vi "GetEntryGoToItem.vi"(3 "error in (no error)":errorcluster, 4 "Return Parameter":u8(ring) items=["Value", "Minimum", "Maximum"], 5 "Element":i16=1 min=1, 6 "VISA resource name":refnum<visa-resource-name>) -> (0 "error out":errorcluster, 1 "Item (N)":u32, 2 "VISA resource name out":refnum<visa-resource-name>)   [LabVIEW 2020, in "Active Technologies AWG3000.lvlib"]
uses:
  Active Technologies AWG3000.lvlib
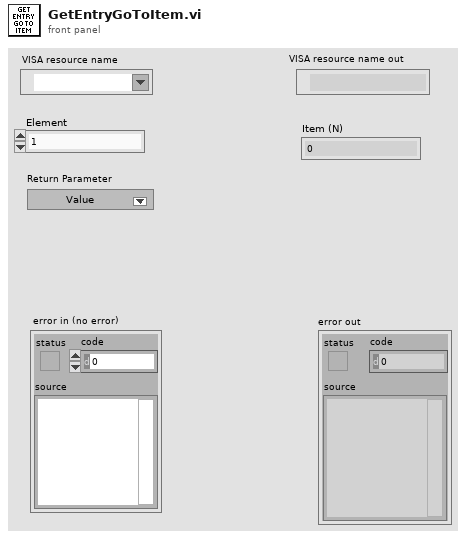
[diagram p1: front panel]
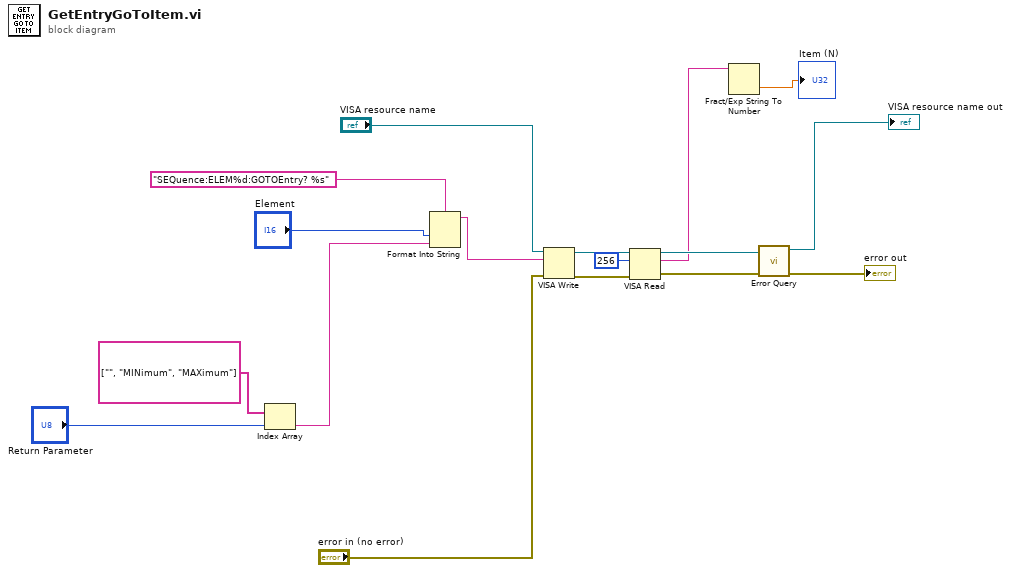
[diagram p0: block diagram]
diagram:
  n1 = Index Array(array=string[] ["", "MINimum", "MAXimum"], index="Return Parameter") -> (element=w2:string)
  n2 = Format Into String(format string="SEQuence:ELEM%d:GOTOEntry? %s" ("write buffer"), "Element", w2) -> (resulting string=w1:string)  [unwired: 2 in, 1 out]
  n3 = VISA Write(VISA resource name="VISA resource name", write buffer=w1, error in (no error)="error in (no error)") -> (VISA resource name out=w12:refnum<visa-resource-name>, error out=w11:errorcluster)  [unwired: 1 out]
  n4 = VISA Read(VISA resource name=w12, byte count=u32 256, error in (no error)=w11) -> (VISA resource name out=w9:refnum<visa-resource-name>, read buffer=w5:string, error out=w8:errorcluster)  [unwired: 1 out]
  n5 = Fract/Exp String To Number(string=w5) -> (number=→"Item (N)":dbl)  [unwired: 3 in, 1 out]
  n6 = call "Error Query.vi"("error in (no error)"=w8, "VISA resource name"=w9) -> ("error out"=→"error out":errorcluster, "VISA resource name out"=→"VISA resource name out":refnum<visa-resource-name>)  [unwired: 6 in, 2 out]
